vi "Read DC Voltage.vi"(1 "Volt Delay":u32=400, 2 "Address":string="24") -> (0 "Voltage":dbl format="%.5e")   [LabVIEW 2013]
panel:
  out "Data":string
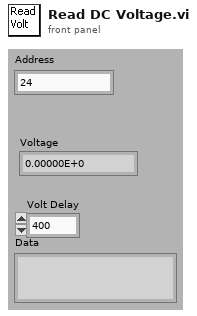
[diagram p1: front panel]
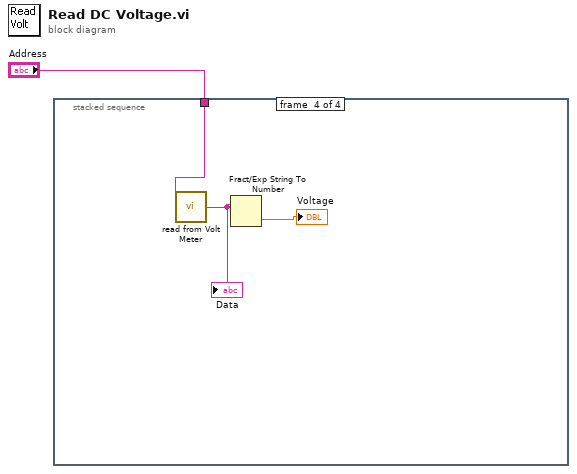
[diagram p0: block diagram]
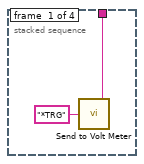
[diagram p2: hidden frame]
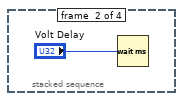
[diagram p3: hidden frame]
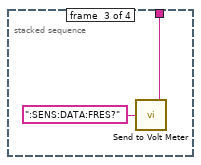
[diagram p4: hidden frame]
diagram:
  n1 = stacked-sequence {
    tunnel: "Address" -> [w3 _ w6 w9]
    frame #0 {
      n2 = call "Send to Volt Meter.vi"("Address"=w3, "Data"="*TRG") -> ()
    }
    frame #1 {
      n3 = Wait (ms)(milliseconds to wait="Volt Delay") -> ()  [unwired: 1 out]
    }
    frame #2 {
      n4 = call "Send to Volt Meter.vi"("Address"=w6, "Data"=":SENS:DATA:FRES?") -> ()
    }
    frame #3 {
      n5 = call "read from Volt Meter.vi"("Address"=w9) -> ("Data"=w7:string)
      "Data" <- w7
      n6 = Fract/Exp String To Number(string=w7) -> (number=→"Voltage":dbl)  [unwired: 3 in, 1 out]
    }
  }
